vi "Read meta data.vi"(8 "error in":errorcluster, 9 "timeout ms (25000)":i32=25000, 11 "connection ID":refnum<k5>) -> (0 "error out":errorcluster, 3 "Connection Info":T1)   [LabVIEW 2021]
uses:
  Connection Info.ctl
panel:
  out "Meta data":string[](array[string])
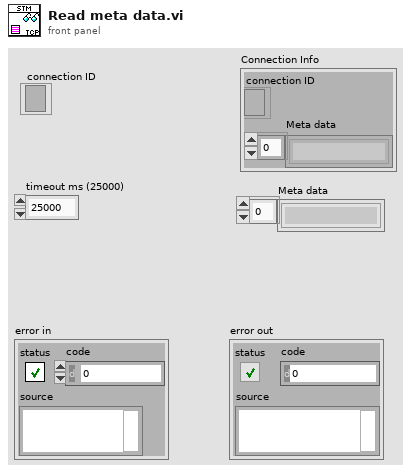
[diagram p1: front panel]
types:
  T1 = typedef "Connection Info.ctl" = cluster{"connection ID":refnum<k5>, "Meta data":string[]}
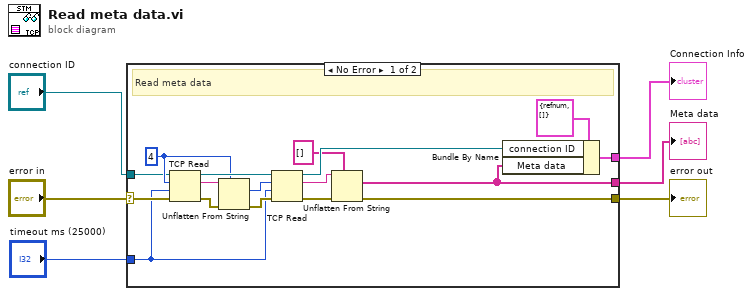
[diagram p0: block diagram]
diagram:
  n1 = case shown="No Error" "error in" {
    selector: "error in" -> [w16 w24]
    tunnel: "connection ID" -> [w14 _]
    tunnel: "timeout ms (25000)" -> [w7 _]
    tunnel: [w12 _] -> w2
    tunnel: [w11 w24] -> w3
    tunnel: [w10 _] -> w1
    frame No Error {
      w15 = 4 ("bytes to read")
      # "Read meta data"
      n2 = TCP Read(connection ID=w14, bytes to read=w15, error in (no error)=w16, 9:w7) -> (connection ID out=w23:refnum<k5>, data out=w20:string, error out=w17:errorcluster)  [unwired: 1 out]
      n3 = Unflatten From String(type=w15, binary string=w20, error in (no error)=w17) -> (value=w18:i32, error out=w19:errorcluster)  [unwired: 3 out]
      n4 = TCP Read(connection ID=w23, bytes to read=w18, error in (no error)=w19, 9:w7) -> (connection ID out=w13:refnum<k5>, data out=w22:string, error out=w21:errorcluster)  [unwired: 1 out]
      n5 = Unflatten From String(type=string[] [] ("Meta data"), binary string=w22, error in (no error)=w21) -> (value=w10:string[], error out=w11:errorcluster)  [unwired: 3 out]
      n6 = Bundle By Name(cluster=T1 {"connection ID"=refnum, "Meta data"=[]} ("Connection Info"), "connection ID"=w13, "Meta data"=w10) -> (w12:T1)
    }
    frame Error {
    }
  }
  "error out" <- w3
  "Connection Info" <- w2
  "Meta data" <- w1
